vi "InstantiateMicronTemplate.vi"() -> ()   [LabVIEW 2019]
uses:
  <vilib>/SLL Toolkit/SLL Scripting/_Typedefs/Rename Item Cluster.ctl
  <vilib>/SLL Toolkit/SLL Scripting/SLL Scripting.lvlib
  <vilib>/SLL Toolkit/SLL File IO/SLL File IO.lvlib
panel:
  in  "New Microservice Name":string
  out "error out":errorcluster
  in  "Micron Template Project Path":path=path "../Templates/MicronTemplate.lvproj"
  in  "Root Directory":path
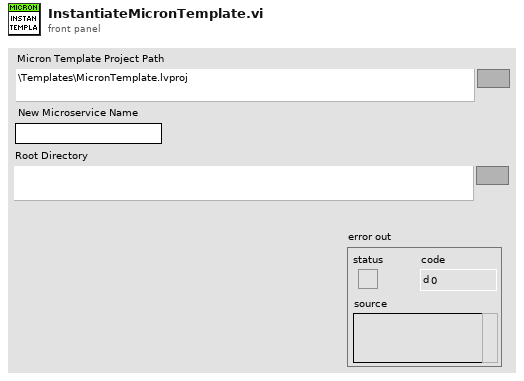
[diagram p1: front panel]
types:
  T1 = typedef "SLL Scripting.lvlib/Rename Item Cluster.ctl" = cluster{"Existing":string, "Rename As":string}
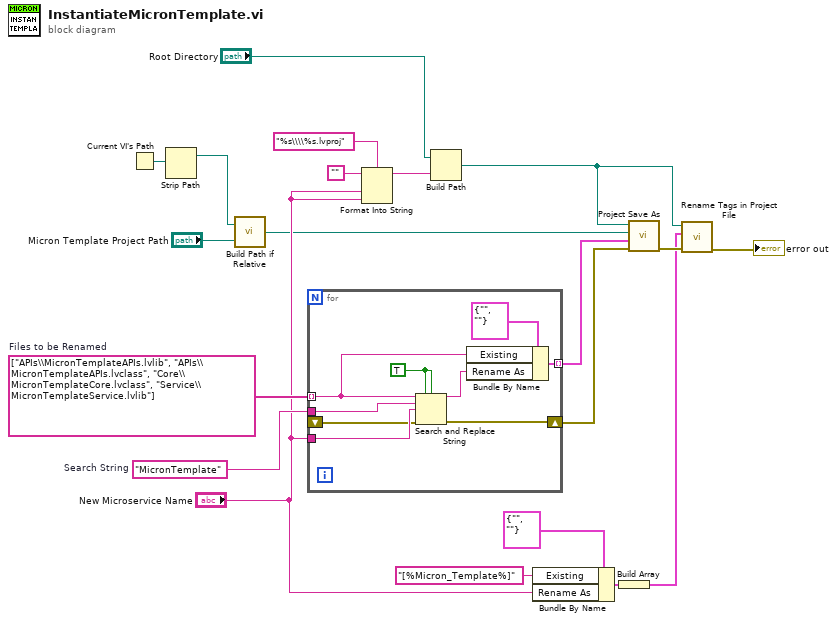
[diagram p0: block diagram]
diagram:
  w19 = "MicronTemplate"  # Search String
  w20 = string[] ["APIs\\MicronTemplateAPIs.lvlib", "APIs\\MicronTemplateAPIs.lvclass", "Core\\MicronTemplateCore.lvclass", "Service\\MicronTemplateService.lvlib"]  # Files to be Renamed
  n1 = Current VI's Path() -> (path=w4:path)
  n2 = Strip Path(path=w4) -> (stripped path=w3:path)  [unwired: 1 out]
  n3 = call <vilib>:"Build Path if Relative.vi"("Relative or Absolute Path"="Micron Template Project Path", "Base Path"=w3) -> ("Path Out"=w2:path)
  n4 = for {
    tunnel: w20 -> [w25] mode=indexing
    tunnel: w19 -> [w29]
    tunnel: "New Microservice Name" -> [w28]
    tunnel: [w23] -> w18 mode=indexing
    shift-right: [w22] -> w17
    shift-left: _ -> [w21]
    w27 = TRUE ("replace all? (F)")
    n5 = Search and Replace String(replace all?=w27, case sensitive?=w27, input string=w25, search string=w29, replace string=w28, error in=w21) -> (result string=w24:string, error out=w22:errorcluster)  [unwired: 2 in, 2 out]
    n6 = Bundle By Name(cluster=T1 {"Existing"="", "Rename As"=""} ("Rename Item"), "Existing"=w25, "Rename As"=w24) -> (w23:T1)
  }
  n7 = Format Into String(format string="%s\\\\%s.lvproj", initial string="", "New Microservice Name", "New Microservice Name") -> (resulting string=w15:string)  [unwired: 1 in, 1 out]
  n8 = Build Path(base path="Root Directory", name or relative path=w15) -> (appended path=w10:path)
  n9 = Bundle By Name(cluster=T1 {"Existing"="", "Rename As"=""} ("Rename Item"), "Existing"="[%Micron_Template%]", "Rename As"="New Microservice Name") -> (w6:T1)
  n10 = Build Array(w6) -> (w5:T1[])
  n11 = call <vilib>:"Project Save As.vi"("error in (no error)"=w17, "Rename Paths[]"=w18, "Existing Project Path"=w2, "New Project Path"=w10) -> ("error out"=w12:errorcluster)  [unwired: 7 in]
  n12 = call <vilib>:"Rename Tags in Project File.vi"("error in (no error)"=w12, "Rename Tags[]"=w5, "Project Path"=w10) -> ("error out"=→"error out":errorcluster)  [unwired: 7 in, 1 out]
